vi "Intake.vi"   [LabVIEW 2020]
uses:
  <vilib>/Rock Robotics/WPI/Solenoid/WPI_SolenoidValue.ctl
  <vilib>/Rock Robotics/WPI/Utilities/WPI_GetSetVariantRefNum.vi
  <vilib>/Rock Robotics/WPI/Solenoid/WPI_SolenoidGetEnum.vi
  <vilib>/Rock Robotics/WPI/Solenoid/WPI_SolenoidSetEnum.vi
types:
  T1 = typedef "WPI_DigitalInputDevRef.ctl" = cluster{"DevStatus":errorcluster, "DIO Channel":T2}
  T2 = typedef "FPGA_DIOChannel.ctl" = enum8{"DIO 0", "DIO 1", "DIO 2", "DIO 3", "DIO 4", "DIO 5", "DIO 6", "DIO 7", "DIO 8", "DIO 9", "DIO MXP 0", "DIO MXP 1", "DIO MXP 2", "DIO MXP 3", "DIO MXP 4", "DIO MXP 5", "DIO MXP 6", "DIO MXP 7", "DIO MXP 8", "DIO MXP 9", "DIO MXP 10", "DIO MXP 11", "DIO MXP 12", "DIO MXP 13", "DIO MXP 14", "DIO MXP 15", "SPI Port CS1", "SPI Port CS2", "SPI Port CS3", "SPI Port MISO", "SPI Port MOSI", "Invalid"}
  T3 = typedef "WPI_JoystickDevRef.ctl" = cluster{"Device":T4}
  T4 = typedef "WPI_JoystickDeviceEnum.ctl" = enum16{"USB 0", "USB 1", "USB 2", "USB 3", "USB 4", "USB 5"}
  T5 = typedef "WPI_SolenoidValue.ctl" = enum16{"Off", "On", "Forward", "Reverse"}
  T6 = typedef "WPI_SolenoidDevRef.ctl" = cluster{"DevStatus":errorcluster, "Pneumatics Control Module":u8, "Forward Solenoid Channel":T7, "Reverse Solenoid Channel":T7}
  T7 = typedef "WPI_SolenoidChannel.ctl" = enum8{"Solenoid 0", "Solenoid 1", "Solenoid 2", "Solenoid 3", "Solenoid 4", "Solenoid 5", "Solenoid 6", "Solenoid 7", "Solenoid 8", "Solenoid 9", "Solenoid 10", "Solenoid 11", "Solenoid 12", "Solenoid 13", "Solenoid 14", "Solenoid 15", "Invalid"}
  T8 = typedef "WPI_MotorControlDeviceRef.ctl" = cluster{"DeviceStatus":errorcluster, "Type":T9, "PWM":cluster{"PWM Channel":T10, "DeadBand":T11}, "CAN":cluster{"Device Number":u8, "SetOutput VI Ref":variant, "GetOutput VI Ref":variant, "Enable VI Ref":variant, "Disable VI Ref":variant, "Data":variant}, "Invert":bool, "DIO PWM":cluster{"PWM \"Enable\" Channel":T10, "DIOChannel":T2, "PWM Rate":dbl}}
  T9 = typedef "WPI_MotorControlType.ctl" = enum16{"PWM", "CAN", "DIO PWM"}
  T10 = typedef "FPGA_DIOPWMChannel.ctl" = enum8{"PWM 0", "PWM 1", "PWM 2", "PWM 3", "PWM 4", "PWM 5", "PWM 6", "PWM 7", "PWM 8", "PWM 9", "PWM MXP 0", "PWM MXP 1", "PWM MXP 2", "PWM MXP 3", "PWM MXP 4", "PWM MXP 5", "PWM MXP 6", "PWM MXP 7", "PWM MXP 8", "PWM MXP 9", "Invalid"}
  T11 = typedef "WPI_PWMDeadband.ctl" = cluster{"Name":string, "maxPositivePwm":i32, "minPositivePwm":i32, "centerPwm":i32, "maxNegativePwm":i32, "minNegativePwm":i32, "angularRange":u16}
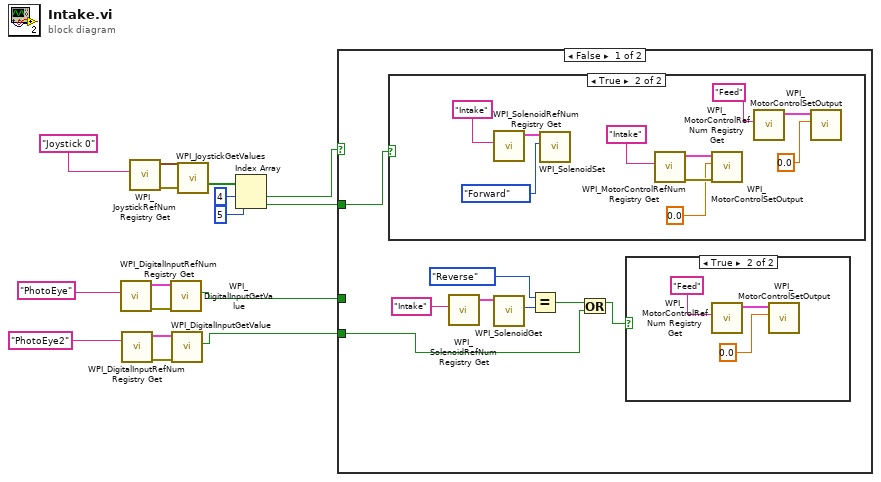
[diagram p0: block diagram]
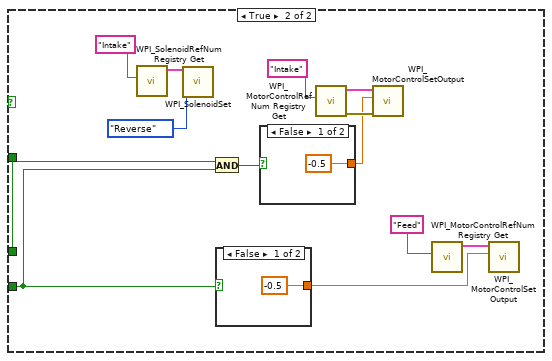
[diagram p4: hidden frame]
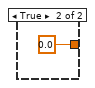
[diagram p5: hidden frame]
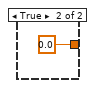
[diagram p6: hidden frame]
diagram:
  n1 = call <vilib>:"WPI_DigitalInputRefNum Registry Get.vi"("refnum name"="PhotoEye") -> ("error out"=w9:errorcluster, "DigitalInputDevRef"=w8:T1)  [unwired: 9 in]
  n2 = call <vilib>:"WPI_DigitalInputRefNum Registry Get.vi"("refnum name"="PhotoEye2") -> ("error out"=w6:errorcluster, "DigitalInputDevRef"=w5:T1)  [unwired: 9 in]
  n3 = call <vilib>:"WPI_JoystickRefNum Registry Get.vi"("refnum name"="Joystick 0") -> ("error out"=w14:errorcluster, "JoystickDevRef"=w15:T3)  [unwired: 1 in, 8 out]
  n4 = call <vilib>:"WPI_DigitalInputGetValue.vi"("error in (no error)"=w9, "DigitalInputDevRef"=w8) -> ("Value"=w7:bool)  [unwired: 7 in, 2 out]
  n5 = call <vilib>:"WPI_DigitalInputGetValue.vi"("error in (no error)"=w6, "DigitalInputDevRef"=w5) -> ("Value"=w1:bool)  [unwired: 7 in, 2 out]
  n6 = call <vilib>:"WPI_JoystickGetValues.vi"("error in (no error)"=w14, "JoystickDevRef"=w15) -> ("Buttons"=w13:bool[])  [unwired: 5 in, 4 out]
  n7 = Index Array(array=w13, index #1=4 ("index"), index #2=5 ("index")) -> (element #1=w10:bool, element #2=w4:bool)
  n8 = case shown="False" w10 {
    tunnel: w7 -> [_ w50]
    tunnel: w1 -> [w17 w39]
    tunnel: w4 -> [w24 _]
    frame False {
      n9 = case shown="True" w24 {
        frame False {
        }
        frame True {
          n10 = call <vilib>:"WPI_SolenoidRefNum Registry Get.vi"("refnum name"="Intake") -> ("SolenoidDevRef"=w35:T6)  [unwired: 9 in, 1 out]
          n11 = call-poly <vilib>:"WPI_SolenoidSet.vi"("Value"=WPI_SolenoidValue."Forward", "SolenoidDevRef"=w35) -> ()  [unwired: 8 in, 2 out]
          n12 = call <vilib>:"WPI_MotorControlRefNum Registry Get.vi"("refnum name"="Intake") -> ("error out"=w36:errorcluster, "MotorControlDevRef"=w37:T8)  [unwired: 9 in]
          n13 = call <vilib>:"WPI_MotorControlSetOutput.vi"("error in (no error)"=w36, "Output"=0.0, "MotorControlDevRef"=w37) -> ()  [unwired: 6 in, 3 out]
          n14 = call <vilib>:"WPI_MotorControlRefNum Registry Get.vi"("refnum name"="Feed") -> ("MotorControlDevRef"=w29:T8)  [unwired: 9 in, 1 out]
          n15 = call <vilib>:"WPI_MotorControlSetOutput.vi"("Output"=0.0, "MotorControlDevRef"=w29) -> ()  [unwired: 7 in, 3 out]
        }
      }
      n16 = call <vilib>:"WPI_SolenoidRefNum Registry Get.vi"("refnum name"="Intake") -> ("SolenoidDevRef"=w22:T6)  [unwired: 9 in, 1 out]
      n17 = call-poly <vilib>:"WPI_SolenoidGet.vi"("SolenoidDevRef"=w22) -> ("Value"=w23:T5)  [unwired: 8 in, 2 out]
      n18 = Equal?(x=WPI_SolenoidValue."Reverse", y=w23) -> (x = y?=w19:bool)
      n19 = Or(x=w19, y=w17) -> (x .or. y?=w18:bool)
      n20 = case shown="True" w18 {
        frame False {
        }
        frame True {
          n21 = call <vilib>:"WPI_MotorControlRefNum Registry Get.vi"("refnum name"="Feed") -> ("MotorControlDevRef"=w27:T8)  [unwired: 9 in, 1 out]
          n22 = call <vilib>:"WPI_MotorControlSetOutput.vi"("Output"=0.0, "MotorControlDevRef"=w27) -> ()  [unwired: 7 in, 3 out]
        }
      }
    }
    frame True {
      n23 = call <vilib>:"WPI_SolenoidRefNum Registry Get.vi"("refnum name"="Intake") -> ("SolenoidDevRef"=w49:T6)  [unwired: 9 in, 1 out]
      n24 = call-poly <vilib>:"WPI_SolenoidSet.vi"("Value"=WPI_SolenoidValue."Reverse", "SolenoidDevRef"=w49) -> ()  [unwired: 8 in, 2 out]
      n25 = And(x=w50, y=w39) -> (x .and. y?=w43:bool)
      n26 = case shown="False" w39 {
        tunnel: [-0.5 ("Output") 0.0 ("Output")] -> w41
        frame False {
        }
        frame True {
        }
      }
      n27 = case shown="False" w43 {
        tunnel: [-0.5 ("Output") 0.0 ("Output")] -> w42
        frame False {
        }
        frame True {
        }
      }
      n28 = call <vilib>:"WPI_MotorControlRefNum Registry Get.vi"("refnum name"="Intake") -> ("error out"=w45:errorcluster, "MotorControlDevRef"=w44:T8)  [unwired: 9 in]
      n29 = call <vilib>:"WPI_MotorControlSetOutput.vi"("error in (no error)"=w45, "Output"=w42, "MotorControlDevRef"=w44) -> ()  [unwired: 6 in, 3 out]
      n30 = call <vilib>:"WPI_MotorControlRefNum Registry Get.vi"("refnum name"="Feed") -> ("MotorControlDevRef"=w40:T8)  [unwired: 9 in, 1 out]
      n31 = call <vilib>:"WPI_MotorControlSetOutput.vi"("Output"=w41, "MotorControlDevRef"=w40) -> ()  [unwired: 7 in, 3 out]
    }
  }
